vi "Input_Value_Dialog.vi"(0 "Message to user":string) -> (1 "Value received":dbl format="%.2f", 2 "Ok Out":bool)   [LabVIEW 2022 SP3]
uses:
  <vilib>/regexp/Match Regular Expression.xnode
panel:
  out "UserMessageDisplay":string
  in  "OK":bool
  in  "Cancel":bool
  in  "Value":dbl format="%.2f"
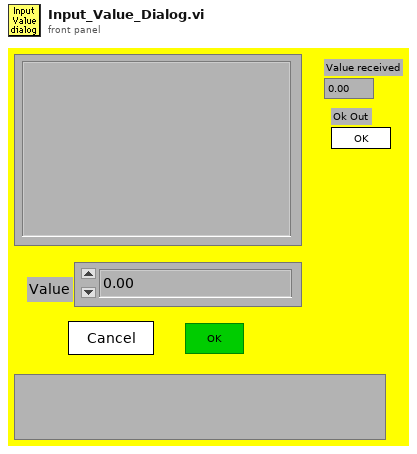
[diagram p1: front panel]
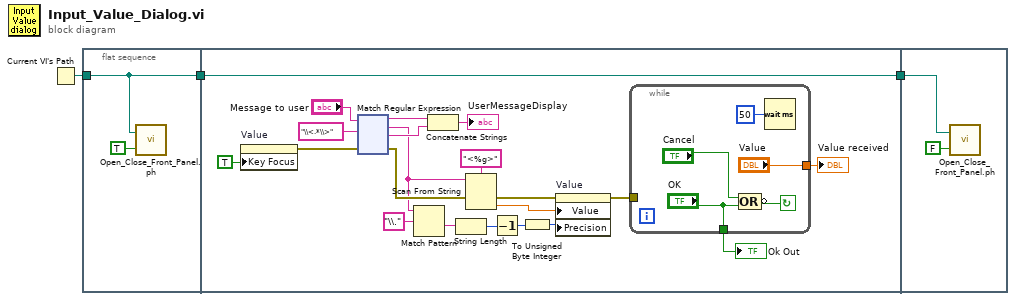
[diagram p0: block diagram]
diagram:
  n1 = Current VI's Path() -> (path=w3:path)
  n2 = flat-sequence {
    tunnel: w3 -> [w5]
    tunnel: [w5] -> w2
    tunnel: w2 -> [w6]
    tunnel: [w6] -> w1
    tunnel: w1 -> [w150]
    frame #0 {
      n3 = call "Open_Close_Front_Panel.ph.vi"("openWindow (T)"=TRUE ("Front Panel Window:Open"), "VI path"=w5) -> ()  [unwired: 1 in, 1 out]
    }
    frame #1 {
      n4 = property on="Value" class="DigNum (strict)"("Key Focus"=TRUE) -> (error out=w20:errorcluster)  [unwired: 2 in, 1 out]
      n5 = xnode "Match Regular Expression"("input string"="Message to user", "regular expression"="\\<.*\\>", "error in"=w20) -> ("before match"=w16:string, "whole match"=w13:string, "after match"=w15:string, "error out"=w19:errorcluster)  [unwired: 3 in, 1 out]
      n6 = Match Pattern(string=w13, regular expression="\\.") -> (after substring=w11:string)  [unwired: 1 in, 3 out]
      n7 = Concatenate Strings(w16, w15) -> (→"UserMessageDisplay":string)
      n8 = String Length(string=w11) -> (length=w10:i32)
      n9 = Scan From String(format string="<%g>", input string=w13, error in=w19) -> (error out=w18:errorcluster, output 1=w14:dbl)  [unwired: 2 in, 2 out]
      n10 = Decrement(x=w10) -> (x-1=w9:i32)
      n11 = To Unsigned Byte Integer(number=w9) -> (unsigned 8bit integer=w8:u8)
      n12 = property on="Value" class="DigNum (strict)"(error in=w18, "Value"=w14, "Precision"=w8) -> (error out=w17:errorcluster)  [unwired: 1 in, 1 out]
      n13 = while {
        tunnel: ["OK"] -> w24
        tunnel: ["Value"] -> w26
        tunnel: w17 -> [_]
        stop <- w147 continue-if-true
        n14 = Compound Arithmetic op=OR("Cancel", "OK") -> (invert w147:bool)
        n15 = Wait (ms)(milliseconds to wait=u32 50) -> ()  [unwired: 1 out]
      }
      "Value received" <- w26
      "Ok Out" <- w24
    }
    frame #2 {
      n16 = call "Open_Close_Front_Panel.ph.vi"("openWindow (T)"=FALSE ("Front Panel Window:Open"), "VI path"=w150) -> ()  [unwired: 1 in, 1 out]
    }
  }
